vi "PH_Timing.PC link SRDG Rate Info.vi"(0 "i ref in":refnum<vi>, 1 "data":i8[](array[numeric]), 2 "Service Name":string="N/A", 3 "typeDescriptor":string="D:N", 4 "no link":bool, 5 "error in":errorcluster) -> (14 "i ref out":refnum<vi>, 19 "error out":errorcluster)   [LabVIEW 2014, in "PH_Timing.lvlib"]
doc: "This VI writes the incoming information to own attributes and sets GUI elements."
uses:
  PH_Timing.lvlib
  PH_Basics/PH_Common/PH_Common.lvlib
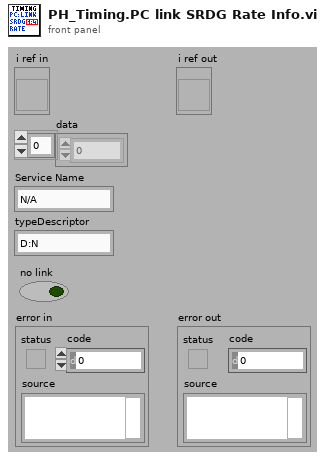
[diagram p1: front panel]
types:
  T1 = typedef "PH_Timing.lvlib/PH_Timing.i attribute.ctl" = cluster{"Sequencer":cluster{"linked?":bool, "Proc State":string, "Ref State":refnum<vi>}, "Gate Generator":cluster{"GD":cluster{"Device Status":T2, "linked?":bool}, "Settings":T3, "GUI Ref":refnum<vi>}, "Interlock Bypass":cluster{"Instancename":string, "Switch linked?":bool, "Device Status":T2, "Ref Status":refnum<vi>}, "Roughtuner":cluster{"Settings":T4, "GUI Ref":refnum<vi>, "GD":cluster{"Device Status":T2, "linked?":bool}}, "0,5Hz Gater":cluster{"Settings":T5, "GUI Ref":refnum<vi>, "GD":cluster{"Device Status":T2, "linked?":bool}}, "Slow Trigger":cluster{"Settings":T6, "GUI Ref":refnum<vi>, "Service ID Delay":i32, "Service ID Ext Trig":i32, "Wanted Settings":T6}, "Timing Mode":cluster{"Mode":T7, "GUI Ref":refnum<vi>, "Service ID T2":i32, "Service ID Mode":i32, "Wanted Mode":T7}, "ns Generator":cluster{"Settings":T8, "ns Generator Settings":refnum<vi>, "GD":cluster{"Device Status":T2, "linked?":bool}}, "Phase FEs":cluster{"Settings":T11, "GUI Ref":refnum<vi>, "Service ID Phase":i32, "Wanted Settings":T11}, "GD GUI Refs":refnum<vi>[], "Heads":T12[], "GUI Ref Delete":refnum<vi>}
  T2 = typedef "PH_StatusHandler.lvlib/PH_StatusHandler.Status.ctl" = i16
  T3 = typedef "PH_Timing.lvlib/PH_Timing.GateGen.ctl" = cluster{"Instance":string, "Channel Gate":i32, "Channel T2":i32, "Width Gate":dbl, "Width T2":dbl, "Delay Gate":dbl, "Delay T2":dbl, "Gate activ":bool, "T2 activ":bool, "System Mode":enum16{"Normal", "Single", "Burst", "Duty Cycle"}}
  T4 = typedef "PH_Timing.lvlib/PH_Timing.Roughtuner.ctl" = cluster{"Instance":string, "Phase PHELIX / UNILAC":cluster{"Channel":u16, "relative to":u16, "Delay [ms]":dbl}, "Pulse Length":cluster{"Channel":u16, "relative to":u16, "Delay [ms]":dbl}, "Trigger":cluster{"externally?":bool, "Rate [Hz]":dbl}}
  T5 = typedef "PH_Timing.lvlib/PH_Timing.0.5HzGater.ctl" = cluster{"Instance":string, "Channel ns FE Delay":i32, "Channel 0.5Hz":i32, "Width ns FE Delay":dbl, "Width 0.5Hz":dbl, "Delay ns FE Delay":dbl, "Delay 0.5Hz":dbl, "ns FE Delay active":bool, "0.5Hz activ":bool, "ns FE Delay inverted":bool, "0.5Hz inverted":bool}
  T6 = typedef "PH_Timing.lvlib/PH_Timing.Slow Trigger Settings.ctl" = cluster{"Delay":dbl, "externally triggered?":bool}
  T7 = typedef "PH_Timing.lvlib/PH_Timing.Timing Mode.ctl" = cluster{"T2":i16, "Modeselector":enum32{"10 Hz", "0.5 Hz", "Shot"}}
  T8 = typedef "PH_Timing.lvlib/PH_Timing.ns Generator.ctl" = cluster{"Instance":string, "Phase fs / ns FE":cluster{"Channel":T9, "Settings":T10}}
  T9 = typedef "Stanford Research DG645 - Driver.lvlib/Channel.ctl" = i32
  T10 = typedef "PH_SRDG645.lvlib/PH_SRDG645.Channel Settings.ctl" = cluster{"Delay [s]":dbl, "relative to":i32}
  T11 = typedef "PH_Timing.lvlib/PH_Timing.Phase FEs.ctl" = cluster{"Phase":dbl}
  T12 = typedef "PH_Timing.lvlib/PH_Timing.PU Data.ctl" = cluster{"linked?":bool, "Data":T13, "GD":cluster{"Device Status":T2, "linked?":bool}, "GUI Ref":refnum<vi>, "PU":T14}
  T13 = typedef "PH_Timing.lvlib/PH_Timing.PU Info.ctl" = cluster{"Act CH?":bool, "GD":string, "CH":i32, "Delay":dbl, "active":bool, "in Use?":bool}
  T14 = typedef "PH_PP_Common.lvlib/PH_PP_Common.PUs.ctl" = enum16{"no Info", "PA-19mm-1", "PA-19mm-2", "PA-45mm-PILC", "PA-45mm-MAIN", "MA-PU-1", "MA-PU-2", "MA-PU-3", "MA-PU-4", "MA-PU-5", "MA-PU-6", "MA-FR", "MA-PILC", "PA-45mm-DP"}
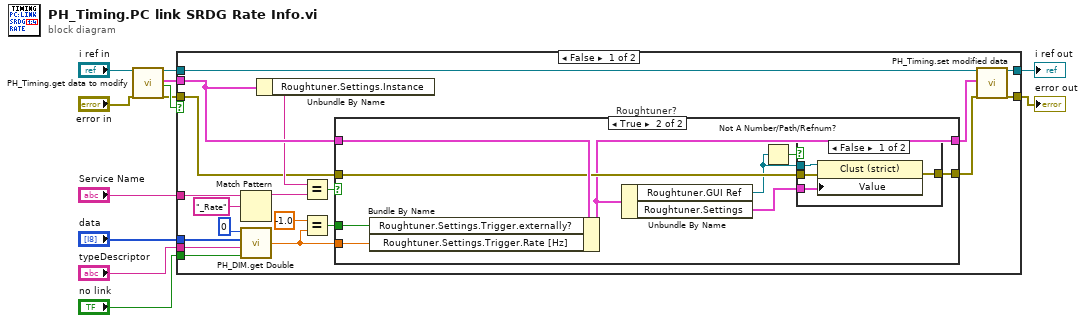
[diagram p0: block diagram]
diagram:
  n1 = call "PH_Timing.get data to modify.vi"("i ref in"="i ref in", "error in (no error)"="error in") -> ("i ref out"=w4:refnum<vi>, "i attribute"=w9:T1, "timed out"=w10:bool, "error out"=w7:errorcluster)  [unwired: 14 in]
  n2 = case shown="False" w10 {
    tunnel: w4 -> [w31 w49]
    tunnel: [w30 w49] -> w5
    tunnel: w7 -> [w20 w48]
    tunnel: [w29 w48] -> w8
    tunnel: w9 -> [w26 _]
    tunnel: "no link" -> [w16 _]
    tunnel: "Service Name" -> [w28 _]
    tunnel: "data" -> [w18 _]
    tunnel: "typeDescriptor" -> [w19 _]
    frame False {
      n3 = Match Pattern(string=w28, regular expression="_Rate") -> (before substring=w22:string)  [unwired: 1 in, 3 out]
      n4 = call "PH_DIM.get Double.vi"("no link"=w16, "typeDescriptor"=w19, "data"=w18, "quality"=0) -> ("Value"=w15:dbl)
      n5 = Unbundle By Name(w26) -> ("Roughtuner.Settings.Instance"=w23:string)
      n6 = Equal?(x=w23, y=w22) -> (x = y?=w21:bool)
      n7 = Equal?(x=-1.0, y=w15) -> (x = y?=w14:bool)
      n8 = case "Roughtuner?" shown="True" w21 {
        tunnel: w26 -> [w33 w42]
        tunnel: [w33 w36] -> w25
        tunnel: w20 -> [w32 w39]
        tunnel: [w32 w35] -> w24
        tunnel: w15 -> [_ w41]
        tunnel: w14 -> [_ w37]
        frame False {
        }
        frame True {
          n9 = Bundle By Name(cluster=w42, "Roughtuner.Settings.Trigger.externally?"=w37, "Roughtuner.Settings.Trigger.Rate [Hz]"=w41) -> (w36:T1)
          n10 = Unbundle By Name(w36) -> ("Roughtuner.GUI Ref"=w34:refnum<vi>, "Roughtuner.Settings"=w40:T4)
          n11 = Not A Number/Path/Refnum?(number/path/refnum=w34) -> (NaN/Path/Refnum?=w38:bool)
          n12 = case shown="False" w38 {
            tunnel: [w46 w47] -> w35
            tunnel: w34 -> [w45 _]
            tunnel: w40 -> [w44 _]
            tunnel: w39 -> [w43 w47]
            frame False {
              n13 = property class="Clust (strict)"(reference=w45, error in=w43, "Value"=w44) -> (error out=w46:errorcluster)  [unwired: 1 out]
            }
            frame True {
            }
          }
        }
      }
      n14 = call "PH_Timing.set modified data.vi"("i ref in"=w31, "i attribute"=w25, "error in (no error)"=w24) -> ("i ref out"=w30:refnum<vi>, "error out"=w29:errorcluster)  [unwired: 15 in]
    }
    frame True {
    }
  }
  "error out" <- w8
  "i ref out" <- w5
